vi "TestAll.vi"() -> ()   [LabVIEW 2015]
uses:
  FPGA3/Limits_In.ctl
  User Interface/Controls/Role ID.ctl
  <vilib>/addons/h5labview/H5F_mode.ctl
  <userlib>/_OpenG.lib/file/file.llb/Build Path - Traditional__ogtk.vi
  <userlib>/_OpenG.lib/array/array.llb/Conditional Auto-Indexing Tunnel (String)__ogtk.vi
  <vilib>/addons/h5labview/polymorph/H5A_read_var.vi
  <userlib>/_OpenG.lib/array/array.llb/Conditional Auto-Indexing Tunnel (I32)__ogtk.vi
  <vilib>/addons/database/_DB Variant To Data/Database Variant To Data.xnode
  <vilib>/addons/h5labview/H5File.lvlib
  <vilib>/addons/h5labview/H5GroupObject.lvlib
  <vilib>/addons/h5labview/H5Attrib.lvlib
panel:
  in  "Mass Error":fxp<+,11,1>=1.0 format="%_4g"
  in  "Velocity Error":fxp<+,11,1>=1.0 format="%_4g"
  in  "Charge Error":fxp<+,11,1>=1.0 format="%_4g"
  out "Fraction Missing":dbl
  out "Stopping Points":u8[][](graph)
  out "Missing Particle Total":i32
  out "Missing Particle Stopping Points":T1(array[cluster])
  out "Missing Particle Totals by Speed":i32[](array[numeric])
  out "Missing Particles by Speed":i32[][](array[numeric])
  out "Total Particles by Speed":i32[](array[numeric])
  out "Particle Total":i32
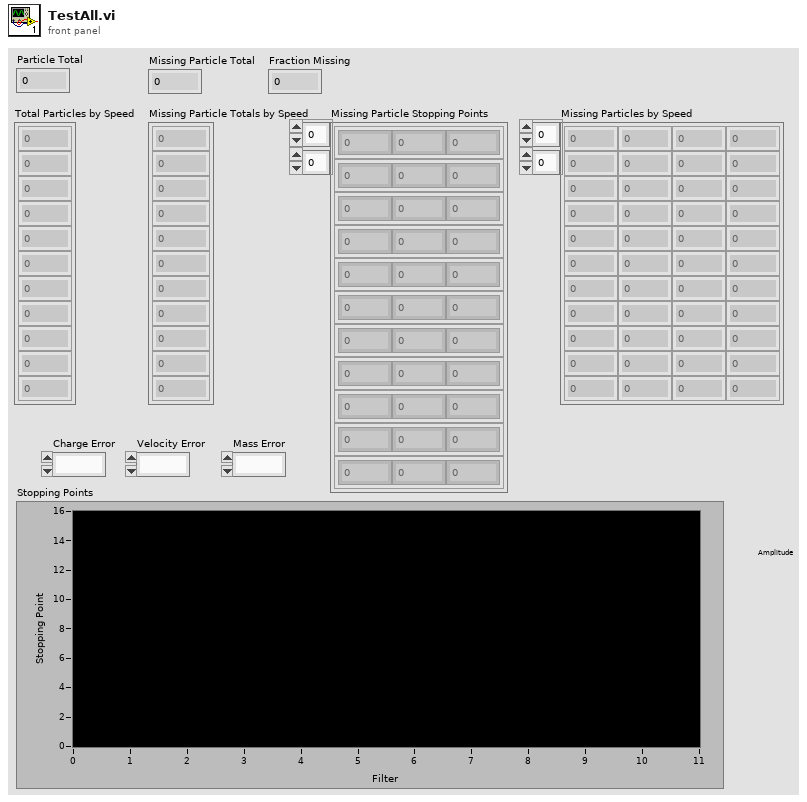
[diagram p1: front panel]
types:
  T1 = cluster{"Max Stop":u8, "Index":i32, "Filter":i32}[][]
  T2 = typedef "Limits_In.ctl" = cluster{"High Charge Limit":fxp<+,32,-41>, "Low Charge Limit":fxp<+,32,-41>, "High Velocity Limit":fxp<+,18,18>, "Low Velocity Limit":fxp<+,18,18>, "High Mass Limit":fxp<+/-,33,-36>, "Low Mass Limit":fxp<+/-,33,-36>, "High Voltage":fxp<+,16,22>}
  T3 = typedef "H5File.lvlib/H5F_mode.ctl" = enum16{"read-only", "read-write", "overwrite", "create new", "open or create"}
  T4 = typedef "Role ID.ctl" = enum16{"First_Detector", "Second_Detector", "Third_Detector", "LeCroy_CH1", "LeCroy_CH2", "LeCroy_CH3", "LeCroy_CH4", "PSU", "DCS 1", "DCS 2"}
  T5 = cluster{"Max Stop":u8, "Index":i32, "Filter":i32}
  T6 = cluster{"Max Stop":u8, "Index":i32, "Filter":i32}[]
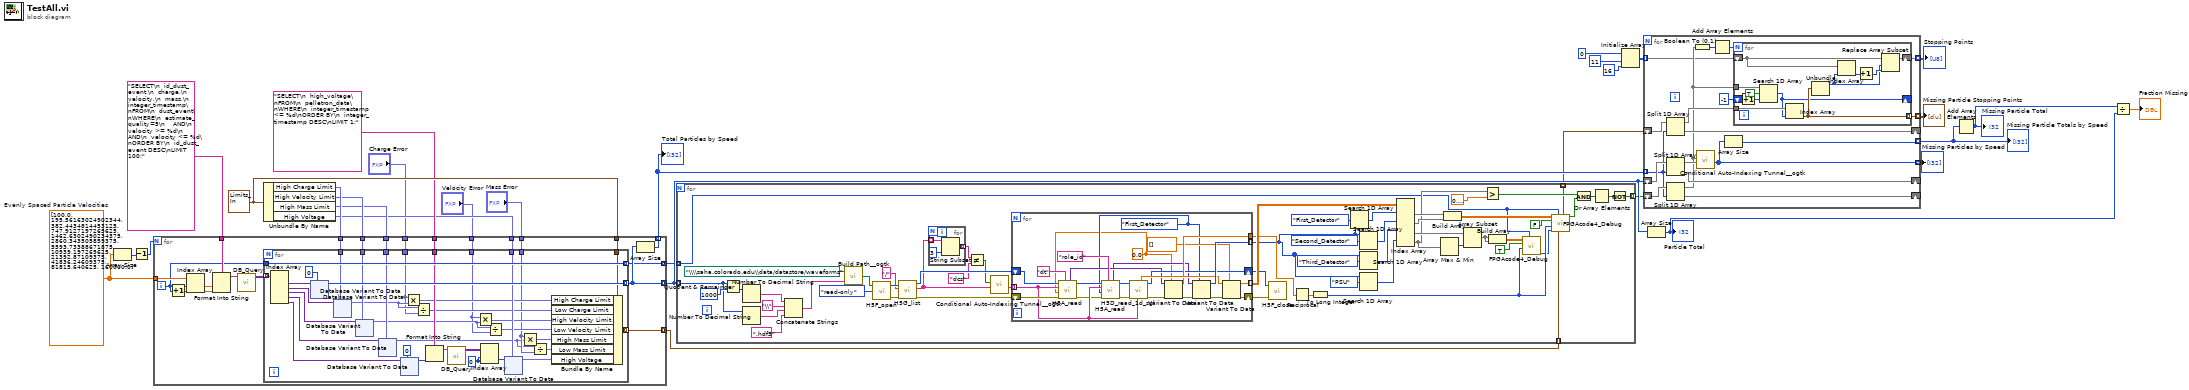
[diagram p0: block diagram]
diagram:
  w7 = T2 {"High Charge Limit"=4.54747350780585e-13, "Low Charge Limit"=0.0, "High Velocity Limit"=262143.0, "Low Velocity Limit"=0.0, "High Mass Limit"=7.27595761248936e-12, "Low Mass Limit"=0.0, "High Voltage"=2200000.0} ("Limits")
  w27 = sgl[] [100.0, 195.56163, 382.44348, 747.9127, 1462.6302, 2860.3435, 5593.734, 10939.197, 21392.871, 41836.246, 81815.64, 160000.0]  # Evenly Spaced Particle Velocities
  n1 = Array Size(array=w27) -> (size(s)=w29:i32)
  n2 = Decrement(x=w29) -> (x-1=w28:i32)
  n3 = Unbundle By Name(w7) -> ("High Charge Limit"=w10:fxp<+,32,-41>, "High Velocity Limit"=w9:fxp<+,18,18>, "High Mass Limit"=w8:fxp<+/-,33,-36>, "High Voltage"=w5:fxp<+,16,22>)
  n4 = for {
    N: w28 -> [_]
    tunnel: "SELECT\n  id_dust_event,\n  charge,\n  velocity,\n  mass,\n  integer_timestamp\nFROM\n  dust_event\nWHERE\n  estimate_quality=5\n    AND\n  velocity >= %d\n    AND\n  velocity <= %d\nORDER BY\n  id_dust_event DESC\nLIMIT 100;" ("Parameterized Query") -> [w51]
    tunnel: [w44] -> w25 mode=concatenating
    tunnel: w27 -> [w47]
    tunnel: [w43] -> w26 mode=indexing
    tunnel: [w41] -> w20 mode=concatenating
    tunnel: w10 -> [w40]
    tunnel: w9 -> [w39]
    tunnel: w8 -> [w38]
    tunnel: w7 -> [w37]
    tunnel: "SELECT\n  high_voltage\nFROM\n  pelletron_data\nWHERE\n  integer_timestamp <= %d\nORDER BY\n  integer_timestamp DESC\nLIMIT 1;" ("Parameterized Query") -> [w36]
    tunnel: w5 -> [w35]
    tunnel: [w34] -> w1 mode=concatenating
    tunnel: "Charge Error" -> [w33]
    tunnel: "Velocity Error" -> [w32]
    tunnel: "Mass Error" -> [w31]
    i -> [w42]
    n5 = Increment(x=w42) -> (x+1=w46:i32)
    n6 = Index Array(array=w47, index #1=w42, index #2=w46) -> (element #1=w49:sgl, element #2=w48:sgl)
    n7 = Format Into String(format string=w51, w49, w48) -> (resulting string=w50:string)  [unwired: 2 in, 1 out]
    n8 = call "DB_Query.vi"("Parameterized Query"=w50) -> ("Results"=w45:variant[][])  [unwired: 8 in, 2 out]
    n9 = for {
      tunnel: [w84] -> w44 mode=indexing
      tunnel: w45 -> [w83] mode=indexing
      tunnel: w42 -> [w82]
      tunnel: [w82] -> w41 mode=indexing
      tunnel: w40 -> [w78]
      tunnel: w39 -> [w77]
      tunnel: w38 -> [w76]
      tunnel: w37 -> [w66]
      tunnel: w36 -> [w72]
      tunnel: w35 -> [w67]
      tunnel: [w65] -> w34 mode=indexing
      tunnel: w33 -> [w60]
      tunnel: w32 -> [w54]
      tunnel: w31 -> [w53]
      w69 = 0 ("disabled index (col)")
      n10 = Index Array(array=w83) -> (element #1=w85:variant, element #2=w81:variant, element #3=w80:variant, element #4=w79:variant, element #5=w75:variant)  [unwired: 5 in]
      n11 = xnode "Database Variant To Data"("database variant"=w85, "type"=0) -> ("data"=w84:i32)  [unwired: 1 in, 1 out]
      n12 = xnode "Database Variant To Data"("database variant"=w81, "type"=w78) -> ("data"=w63:fxp<+,32,-41>)  [unwired: 1 in, 1 out]
      n13 = xnode "Database Variant To Data"("database variant"=w80, "type"=w77) -> ("data"=w59:fxp<+,18,18>)  [unwired: 1 in, 1 out]
      n14 = xnode "Database Variant To Data"("database variant"=w79, "type"=w76) -> ("data"=w52:fxp<+/-,33,-36>)  [unwired: 1 in, 1 out]
      n15 = xnode "Database Variant To Data"("database variant"=w75, "type"=i64 0) -> ("data"=w73:i64)  [unwired: 1 in, 1 out]
      n16 = Multiply(x=w60, y=w63) -> (x*y=w61:fxp<+,43,-40>)
      n17 = Divide(x=w63, y=w60) -> (x/y=w62:fxp<+,43,-31>)
      n18 = Format Into String(format string=w72, w73) -> (resulting string=w71:string)  [unwired: 2 in, 1 out]
      n19 = call "DB_Query.vi"("Parameterized Query"=w71) -> ("Results"=w70:variant[][])  [unwired: 8 in, 2 out]
      n20 = Multiply(x=w54, y=w59) -> (x*y=w56:fxp<+,29,19>)
      n21 = Index Array(array=w70, index (row)=w69, index (col)=w69) -> (element=w68:variant)
      n22 = Divide(x=w59, y=w54) -> (x/y=w55:fxp<+,29,28>)
      n23 = xnode "Database Variant To Data"("database variant"=w68, "type"=w67) -> ("data"=w64:fxp<+,16,22>)  [unwired: 1 in, 1 out]
      n24 = Multiply(x=w53, y=w52) -> (x*y=w57:fxp<+/-,44,-35>)
      n25 = Divide(x=w52, y=w53) -> (x/y=w58:fxp<+/-,44,-26>)
      n26 = Bundle By Name(cluster=w66, "High Charge Limit"=w61, "Low Charge Limit"=w62, "High Velocity Limit"=w56, "Low Velocity Limit"=w55, "High Mass Limit"=w57, "Low Mass Limit"=w58, "High Voltage"=w64) -> (w65:T2)
    }
    n27 = Array Size(array=w44) -> (size(s)=w43:i32)
  }
  "Total Particles by Speed" <- w26
  n28 = for {
    tunnel: [w306] -> w24 mode=indexing
    tunnel: w25 -> [w287] mode=indexing
    tunnel: [w286] -> w22 mode=indexing
    tunnel: w20 -> [w285] mode=indexing
    tunnel: w1 -> [w279] mode=indexing
    n29 = Quotient & Remainder(x=w287, y=1000) -> (floor(x/y)=w290:i32)  [unwired: 1 out]
    n30 = Number To Decimal String(number=w290) -> (decimal integer string=w292:string)  [unwired: 1 in]
    n31 = Number To Decimal String(number=w287) -> (decimal integer string=w294:string)  [unwired: 1 in]
    n32 = Concatenate Strings(w292, "\\" ("string"), w294, ".hdf5" ("string")) -> (w298:string)
    n33 = call-poly <userlib>:"Build Path__ogtk.vi"("name or relative path"=w298, "base path"=path "\\\\saha.colorado.edu\\data/datastore/waveforms") -> ("appended path"=w300:path)
    n34 = call <vilib>:"H5F_open.vi"("mode"=H5F_mode."read-only", "path"=w300) -> ("error out"=w296:errorcluster, "ref"=w297:i32)  [unwired: 2 in]
    n35 = call <vilib>:"H5G_list.vi"("error in (no error)"=w296, "group"="/", "ref"=w297) -> ("error out"=w289:errorcluster, "names"=w280:string[], "ref out"=w288:i32)  [unwired: 1 in, 1 out]
    n36 = for {
      tunnel: w280 -> [w336] mode=indexing
      tunnel: [w335] -> w282 mode=indexing
      n37 = String Subset(string=w336, length (rest)=3 ("length (rest)")) -> (substring=w335:string)  [unwired: 1 in]
    }
    n38 = Not Equal?(x=w282, y="dcs") -> (x != y?=w283:bool[])
    n39 = call-poly <userlib>:"Conditional Auto-Indexing Tunnel__ogtk.vi"("Array in"=w280, "Elements to keep"=w283) -> ("Filtered Array out"=w284:string[])  [unwired: 5 in]
    n40 = for {
      shift-right: [w349] -> w304
      shift-left: w289 -> [w353]
      shift-right: [w347] -> w303
      shift-left: w288 -> [w354]
      tunnel: [w356] -> w320 mode=indexing
      tunnel: [w357] -> w334 mode=indexing
      tunnel: [w352] -> w324
      tunnel: w284 -> [w346] mode=indexing
      w339 = 0.0
      w340 = Role_ID."First_Detector" ("Role ID")
      n41 = call-poly <vilib>:"H5A_read.vi"("attrib_name"="dt", "error in (no error)"=w353, "default"=w339, "obj_name"=w346, "ref"=w354) -> ("error out"=w342:errorcluster, "ref out"=w348:i32, "value"=w344:variant)  [unwired: 2 in]
      n42 = call-poly <vilib>:"H5A_read.vi"("attrib_name"="role_id", "error in (no error)"=w342, "default"=w340, "obj_name"=w346, "ref"=w348) -> ("error out"=w341:errorcluster, "ref out"=w358:i32, "value"=w343:variant)  [unwired: 2 in]
      n43 = call "H5D_read_1d_sgl.vi"("name"=w346, "error in (no error)"=w341, "ref"=w358) -> ("error out"=w338:errorcluster, "ref out"=w347:i32, "data"=w355:sgl[])  [unwired: 4 in]
      n44 = Variant To Data(error in=w338, type=w339, Variant=w344) -> (data=w352:dbl, error out=w350:errorcluster)
      n45 = Variant To Data(error in=w350, type=w340, Variant=w343) -> (data=w356:T4, error out=w359:errorcluster)
      n46 = Variant To Data(error in=w359, type=sgl[] [] ("Data"), Variant=w355) -> (data=w357:sgl[], error out=w349:errorcluster)
    }
    n47 = call <vilib>:"H5F_close.vi"("error in (no error)"=w304, "ref"=w303) -> ()  [unwired: 3 in, 1 out]
    n48 = Reciprocal(x=w324) -> (1/x=w323:dbl)
    n49 = To Long Integer(number=w323) -> (32bit integer=w322:i32)
    n50 = Search 1D Array(1D array=w320, element=Role_ID."First_Detector") -> (index of element=w331:i32)  [unwired: 1 in]
    n51 = Search 1D Array(1D array=w320, element=Role_ID."Second_Detector") -> (index of element=w330:i32)  [unwired: 1 in]
    n52 = Search 1D Array(1D array=w320, element=Role_ID."Third_Detector") -> (index of element=w328:i32)  [unwired: 1 in]
    n53 = Search 1D Array(1D array=w320, element=Role_ID."PSU") -> (index of element=w319:i32)  [unwired: 1 in]
    n54 = Index Array(array=w334, index (row) #1=w331, index (row) #2=w330, index (row) #3=w328, index (row) #4=w319) -> (element #1=w318:sgl[], element #2=w316:sgl[], element #3=w314:sgl[], element #4=w312:sgl[])  [unwired: 4 in]
    n55 = Array Max & Min(array=w312) -> (max index (indices)=w315:i32)  [unwired: 3 out]
    n56 = Build Array(w318, w316) -> (w327:sgl[][])
    n57 = Array Subset(array=w314, length=w315) -> (w313:sgl[])  [unwired: 1 in]
    n58 = Greater?(x=w312, y=sgl 0.1) -> (0:w310:bool[])
    n59 = Build Array(w313, w313) -> (w325:sgl[][])
    n60 = call "FPGAcode4_Debug.vi"("Speed Bracket"=w285, "Clock Speed (Hz)"=w322, "Calibrate"=TRUE, "Detector Waveform In"=w325) -> ("Thresholds out"=w317:i32[])  [unwired: 2 in, 5 out]
    n61 = call "FPGAcode4_Debug.vi"("Limits"=w279, "Speed Bracket"=w285, "Thresholds in"=w317, "Clock Speed (Hz)"=w322, "Calibrate"=FALSE, "Detector Waveform In"=w327) -> ("PSU Response"=w309:bool[], "Max Stop Point"=w286:T5)  [unwired: 4 out]
    n62 = And(x=w310, y=w309) -> (x .and. y?=w308:bool[])
    n63 = Or Array Elements(Boolean array=w308) -> (logical OR=w307:bool)
    n64 = Not(x=w307) -> (.not. x?=w306:bool)
  }
  n65 = Initialize Array(u8 0 ("Stopping Points"), 11 ("dimension size"), 16 ("dimension size")) -> (w15:u8[][])
  n66 = for {
    tunnel: w26 -> [w370] mode=indexing
    shift-right: [w378] -> _
    shift-left: w25 -> [w377]
    shift-right: [w375] -> _
    shift-left: w24 -> [w376]
    tunnel: [w373] -> w23 mode=indexing
    tunnel: [w372] -> w19 mode=indexing
    shift-right: [w369] -> _
    shift-left: w22 -> [w371]
    tunnel: [w366] -> w21 mode=indexing
    tunnel: w15 -> [w362] mode=indexing
    tunnel: [w361] -> w14 mode=indexing
    n67 = Split 1D Array(array=w371, index=w370) -> (first subarray=w368:T6, second subarray=w369:T6)
    n68 = Split 1D Array(array=w377, index=w370) -> (first subarray=w374:i32[], second subarray=w378:i32[])
    n69 = Split 1D Array(array=w376, index=w370) -> (first subarray=w364:bool[], second subarray=w375:bool[])
    n70 = Boolean To (0,1)(Boolean=w364) -> (0, 1=w365:i16[])
    n71 = call-poly <userlib>:"Conditional Auto-Indexing Tunnel__ogtk.vi"("Array in"=w374, "Elements to keep"=w364) -> ("Filtered Array out"=w373:i32[])  [unwired: 5 in]
    n72 = Add Array Elements(numeric array=w365) -> (sum=w363:i16)
    n73 = Array Size(array=w373) -> (size(s)=w372:i32)
    n74 = for {
      N: w363 -> [_]
      tunnel: w368 -> [w387]
      tunnel: w364 -> [w389]
      shift-right: [w380] -> _
      shift-left: -1 ("start index (0)") -> [w390]
      tunnel: [w386] -> w366 mode=indexing
      shift-right: [w381] -> w361
      shift-left: w362 -> [w384]
      n75 = Increment(x=w390) -> (x+1=w379:i32)
      n76 = Search 1D Array(1D array=w389, element=TRUE, start index (0)=w379) -> (index of element=w380:i32)
      n77 = Index Array(array=w387, index=w380) -> (element=w386:T5)
      n78 = Unbundle(w386) -> ("Max Stop"=w382:u8)  [unwired: 2 out]
      n79 = Index Array(array=w384, index=w382) -> (element=w385:u8)
      n80 = Increment(x=w385) -> (x+1=w383:u8)
      n81 = Replace Array Subset(array=w384, new element=w383, index=w382) -> (w381:u8[])
    }
  }
  "Missing Particles by Speed" <- w23
  "Missing Particle Totals by Speed" <- w19
  "Missing Particle Stopping Points" <- w21
  "Stopping Points" <- w14
  n82 = Array Size(array=w25) -> (size(s)=w12:i32)
  "Particle Total" <- w12
  n83 = Add Array Elements(numeric array=w19) -> (sum=w13:i32)
  "Missing Particle Total" <- w13
  n84 = Divide(x=w13, y=w12) -> (x/y=→"Fraction Missing":dbl)
